vi "Set Integration.vi"(8 "error in (no error)":errorcluster, 10 "Integ Count":u32, 11 "Mode":i16) -> (0 "error out":errorcluster)   [LabVIEW 2015, in "Tool Interface.lvlib"]
uses:
  Tool Interface.lvlib
  Tool Typedefs/_Integration Params Cluster--typedef.ctl
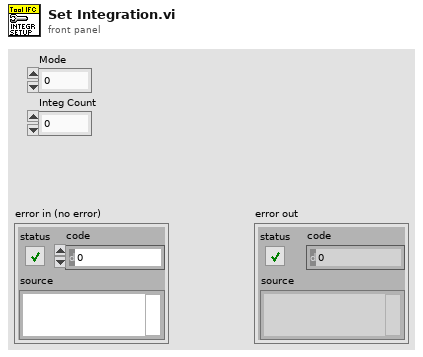
[diagram p1: front panel]
types:
  T1 = typedef "_Integration Params Cluster--typedef.ctl" = cluster{"Mode":i16, "Integ Count":u32}
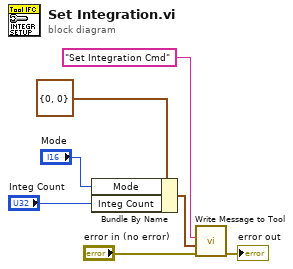
[diagram p0: block diagram]
diagram:
  n1 = Bundle By Name(cluster=T1 {"Mode"=0, "Integ Count"=0} ("_Laser Params Cluster--typedef"), "Mode"="Mode", "Integ Count"="Integ Count") -> (w6:T1)
  n2 = call "Write Message to Tool.vi"("error in (no error)"="error in (no error)", "Message Data"=w6, "Message"="Set Integration Cmd") -> ("error out"=→"error out":errorcluster)  [unwired: 8 in]
